vi "MeasuringDevice.UnInit.vi"(8 "error in (no error)":errorcluster, 11 "LIA.SR810":refnum<class "LIA.SR810.lvclass">) -> (0 "error out":errorcluster, 3 "LIA.SR810 out":refnum<class "LIA.SR810.lvclass">)   [LabVIEW 2017, in "LIA.SR810.lvclass"]
doc: "---------------------------------------------------------------\nJKI State Machine Objects™\nhttp://jki.net/state-machine-objects/\nCopyright (C) 2005-2015, JKI <info@jki.net>\nALL RIGHTS RESERVEDJKI State Machine Objects (SMO) 1.0.0.5\nJKI - JKI\nCopyright (c) 2016, JKI"
uses:
  LIA.SR810.lvclass
  LIA/LIA.lvclass
  <instrlib>/Stanford Research 830/Stanford Research 830.lvlib
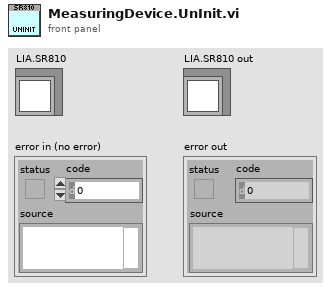
[diagram p1: front panel]
types:
  T1 = cluster{"VISA resource":refnum<visa-resource-name>}
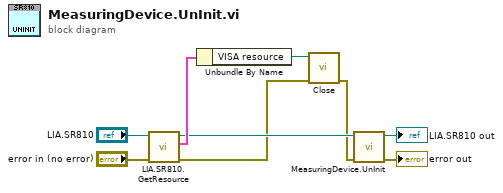
[diagram p0: block diagram]
diagram:
  n1 = call "LIA.SR810.GetResource.vi"("error in (no error)"="error in (no error)", "LIA.SR810 in"="LIA.SR810") -> ("error out"=w2:errorcluster, "Resource"=w5:T1, "LIA.SR810 out"=w3:refnum<class "LIA.SR810.lvclass">)  [unwired: 7 in]
  n2 = Unbundle By Name(w5) -> ("VISA resource"=w4:refnum<visa-resource-name>)
  n3 = call <instrlib>:"Close.vi"("error in (no error)"=w2, "VISA resource name"=w4) -> ("error out"=w1:errorcluster)  [unwired: 9 in]
  n4 = call-parent "MeasuringDevice.UnInit.vi"("error in (no error)"=w1, "MeasuringDevice"=w3) -> ("error out"=→"error out":errorcluster, "MeasuringDevice out"=→"LIA.SR810 out":refnum<class "LIA.SR810.lvclass">)  [unwired: 8 in]
